vi "Help.vi"() -> ()   [LabVIEW 2014, in "Aquisicao de Dados.lvlib"]
uses:
  Aquisicao de Dados.lvlib
panel:
  in  "Tab Control":T1(tab)
  # "Ajuda"
  # "Este programa de por funcionalidade auxiliar na seleção de fontes de dados para o projeto, direcionando a atenção do aluno para o processo de compreensão e analize dos sinais selecionados.\n\nNesta ferramenta você poderá selecionar uma de quatro fontes de dados suportados pelo programa (Simulação LTSpice, Simulação Multisim, Arquivo de Audio .WAV ou diretamente por um dispositivo de entrada de seu computador); selecionar as configurações de importação/aquisição de dados; e pre-visualizar o sinal a ser obtido.\n\nAutoria: Rodrigo Anjos de Souza (rodrigo.anjos.souza@usp.br"
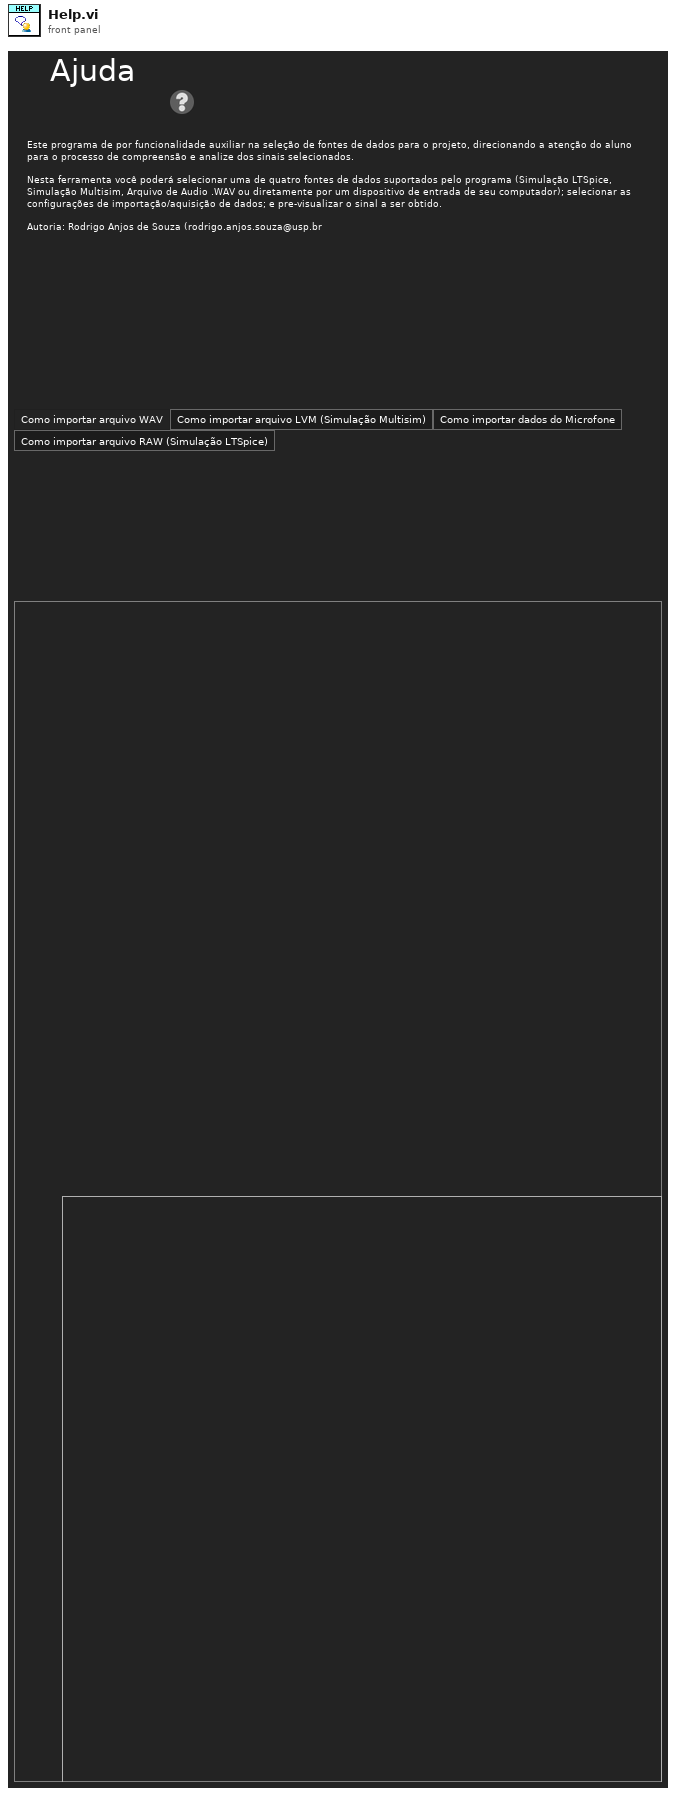
[diagram p1: front panel]
types:
  T1 = enum32{"Como importar arquivo WAV", "Como importar arquivo LVM (Simulação Multisim)", "Como importar dados do Microfone", "Como importar arquivo RAW (Simulação LTSpice)"}
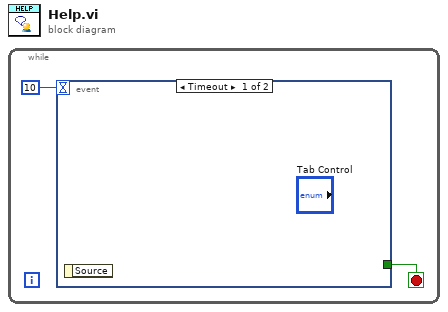
[diagram p0: block diagram]
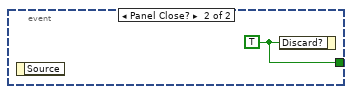
[diagram p2: hidden frame]
diagram:
  n1 = while {
    stop <- w2 stop-if-true
    n2 = event shown="[0] Timeout" {
      selector: _ -> [_ _]
      dyn-events: _ -> [_ _]
      timeout: 10 -> [_ _]
      tunnel: [_ w3] -> w2
      event Timeout {
        n3 = event-data() -> ()  [unwired: 1 in, 1 out]
      }
      event Panel Close? {
        w3 = TRUE ("Discard?")
        n4 = event-data() -> ()  [unwired: 1 in, 1 out]
        n5 = event-data("Discard?"=w3) -> ()  [unwired: 1 in, 1 out]
      }
    }
  }
